vi "Replace All GUIDs.vi"(8 "error in":errorcluster, 10 "xml path":path, 11 "constants vi paths":path[](array[path])) -> (0 "error out":errorcluster)   [LabVIEW 2020, in "GUID Tool.lvlib"]
uses:
  GUID Tool.lvlib
  NationalInstruments.VeriStand.XMLReader
  b6d98739-f8a9-4836-a413-71a9372ff6fb.vi
  b6d98739-f8a9-4836-a413-71a9372ff6fb.vi/e8389a26-e8e5-4d45-8f45-fcb1de2d9257.vi
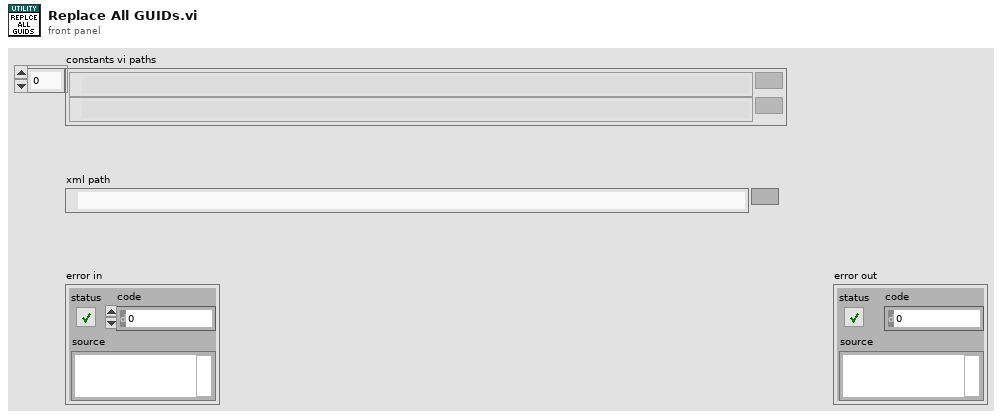
[diagram p1: front panel]
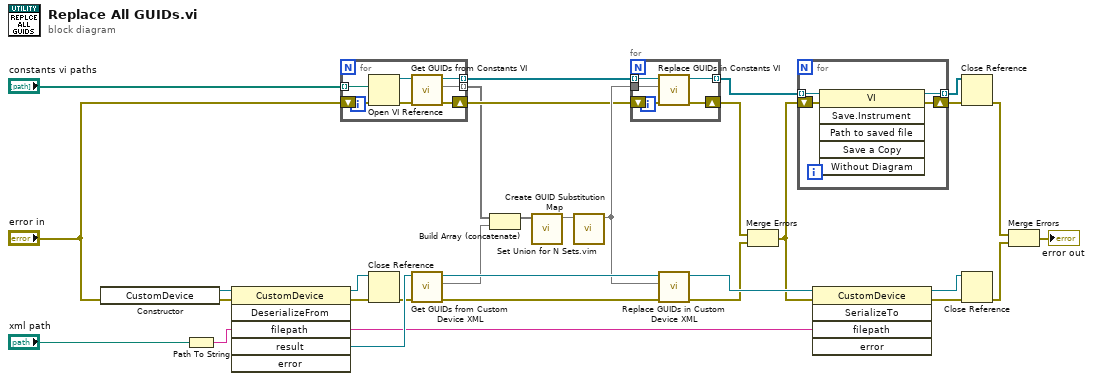
[diagram p0: block diagram]
diagram:
  n1 = constructor class="CustomDevice"(error in="error in") -> (reference out=w29:refnum<k24>, error out=w30:errorcluster)  [unwired: 2 in, 1 out]
  n2 = Path To String(path="xml path") -> (string=w21:string)
  n3 = invoke class="CustomDevice" method="DeserializeFrom"(reference=w29, error in=w30, "filepath"=w21) -> (reference out=w22:refnum<k24>, error out=w23:errorcluster, "result"=w27:refnum<k24>)  [unwired: 3 in, 3 out]
  n4 = for {
    tunnel: "constants vi paths" -> [w38] mode=indexing
    tunnel: [w36] -> w18 mode=indexing
    tunnel: [w33] -> w10 mode=indexing
    shift-right: [w35] -> w12
    shift-left: "error in" -> [w32]
    n5 = Open VI Reference(vi path=w38, error in (no error)=w32) -> (vi reference=w37:refnum<vi>, error out=w34:errorcluster)  [unwired: 4 in]
    n6 = call "Get GUIDs from Constants VI.vi"("error in"=w34, "VI in"=w37) -> ("error out"=w35:errorcluster, "set out"=w33:set{string}, "VI out"=w36:refnum<vi>)  [unwired: 7 in]
  }
  n7 = Close Reference(reference=w22, error in (no error)=w23) -> (error out=w11:errorcluster)
  n8 = call "Get GUIDs from Custom Device XML.vi"("error in"=w11, "CustomDevice in"=w27) -> ("error out"=w13:errorcluster, "set out"=w2:set{string}, "CustomDevice out"=w25:refnum<k24>)  [unwired: 6 in]
  n9 = Build Array (concatenate)(w10, w2) -> (w3:set{string}[])
  n10 = call "Set Union for N Sets.vim"("sets"=w3) -> ("union"=w26:set{string})  [unwired: 10 in]
  n11 = call "Create GUID Substitution Map.vi"("guids"=w26) -> ("guid map"=w17:map{string, string})  [unwired: 10 in]
  n12 = for {
    tunnel: w18 -> [w43] mode=indexing
    tunnel: w17 -> [w42]
    tunnel: [w41] -> w16 mode=indexing
    shift-right: [w39] -> w8
    shift-left: w12 -> [w40]
    n13 = call "Replace GUIDs in Constants VI.vi"("error in"=w40, "guid map"=w42, "VI in"=w43) -> ("error out"=w39:errorcluster, "VI out"=w41:refnum<vi>)  [unwired: 7 in]
  }
  n14 = call "Replace GUIDs in Custom Device XML.vi"("error in"=w13, "guid map"=w17, "CustomDevice in"=w25) -> ("error out"=w9:errorcluster, "CustomDevice out"=w24:refnum<k24>)  [unwired: 6 in]
  n15 = Merge Errors(w8, w9) -> (w7:errorcluster)
  n16 = for {
    tunnel: w16 -> [w47] mode=indexing
    tunnel: [w45] -> w14 mode=indexing
    shift-right: [w46] -> w15
    shift-left: w7 -> [w44]
    n17 = invoke class="VI" method="Save.Instrument"(reference=w47, error in=w44) -> (reference out=w45:refnum<vi>, error out=w46:errorcluster)  [unwired: 4 in, 4 out]
  }
  n18 = invoke class="CustomDevice" method="SerializeTo"(reference=w24, error in=w7, "filepath"=w21) -> (reference out=w19:refnum<k24>, error out=w20:errorcluster)  [unwired: 2 in, 3 out]
  n19 = Close Reference(reference=w14, error in (no error)=w15) -> (error out=w6:errorcluster)
  n20 = Close Reference(reference=w19, error in (no error)=w20) -> (error out=w5:errorcluster)
  n21 = Merge Errors(w6, w5) -> (→"error out":errorcluster)
